vi "TestPVCam_DiskStreaming2.vi"(8 "error in":errorcluster, 10 "Exposure time [ms]":T5=20) -> (0 "error out":errorcluster)   [LabVIEW 2023, in "Photometrics Camera.lvlib"]
uses:
  Photometrics Camera.lvlib
  <userlib>/TPM LabVIEW adapter/SDK/Controls/Exposure Time.ctl
  <userlib>/TPM LabVIEW adapter/SDK/Controls/Frames To Capture.ctl
  <userlib>/TPM LabVIEW adapter/SDK/Controls/Frames Captured.ctl
  <userlib>/TPM LabVIEW adapter/SDK/Controls/Camera Description.ctl
  <userlib>/TPM LabVIEW adapter/PVCAM/PVCAM.lvclass
  <userlib>/TPM LabVIEW adapter/SDK/Controls/All Params IDs.ctl
  <userlib>/TPM LabVIEW adapter/SDK/Controls/Buffer Size.ctl
  <userlib>/TPM LabVIEW adapter/SDK/Controls/Disk Streaming Options.ctl
  <userlib>/TPM LabVIEW adapter/SDK/Controls/Disk Streaming File Name.ctl
  <userlib>/TPM LabVIEW adapter/SDK/Controls/Disk Streaming File Size.ctl
  <userlib>/TPM LabVIEW adapter/SDK/Enum params values/ENUMS/ENUM EXP RES MODES.ctl
  <userlib>/TPM LabVIEW adapter/SDK/Enum params values/RINGS/RING EXPOSURE MODES.ctl
  <userlib>/TPM LabVIEW adapter/SDK/Enum params values/ENUMS/ENUM EXPOSE OUT MODES.ctl
  <userlib>/TPM LabVIEW adapter/SDK/Controls/Acquisition Mode.ctl
  <userlib>/TPM LabVIEW adapter/Camera/Camera.lvclass
panel:
  out "Camera Description":T1
  out "Camera 0 Name":string
  out "Pixels UNS16":u16[](array[numeric])
  out "Disk Streaming Queue Count":u32
  out "Frames Captured":T2
  out "Image":T3(plugin-control)
  in  "Frames To Capture":T4=1000
  out "Disk Streaming Failed":bool
  out "Disk Streaming Dropped Frames":u64
  out "FPS":dbl
  out "Number of cameras":u32
  in  "STOP":bool
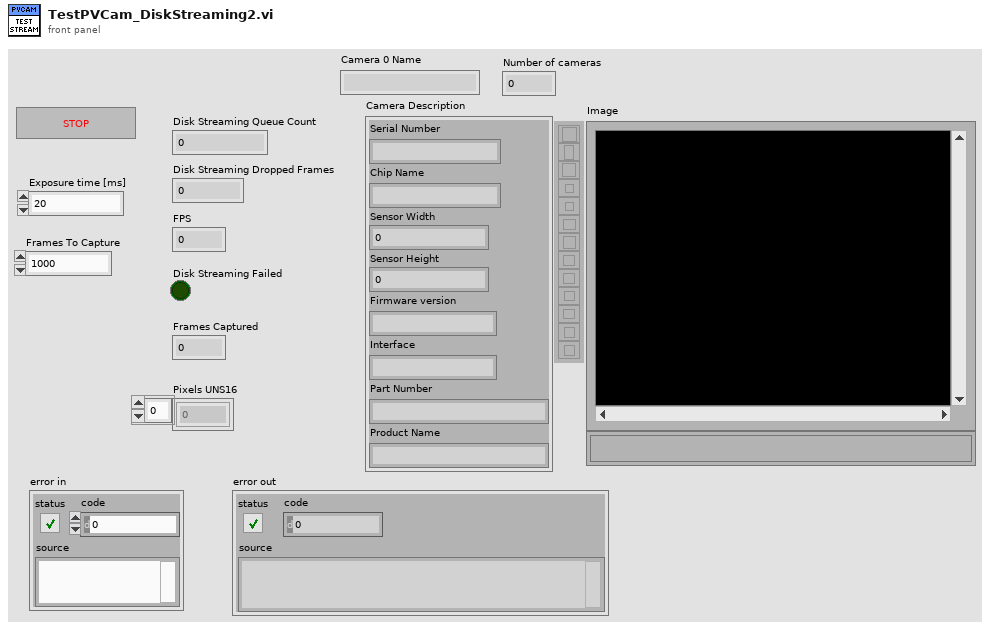
[diagram p1: front panel]
types:
  T1 = typedef "Camera Description.ctl" = cluster{"Serial Number":string, "Chip Name":string, "Sensor Width":u32, "Sensor Height":u32, "Firmware version":string, "Interface":string, "Part Number":string, "Product Name":string}
  T2 = typedef "Frames Captured.ctl" = u64
  T3 = typedef "IMAQ Image.ctl" = refnum<image>
  T4 = typedef "Frames To Capture.ctl" = u32
  T5 = typedef "Exposure Time.ctl" = u32
  T6 = typedef "ENUM EXPOSE OUT MODES.ctl" = enum32{"EXPOSE_OUT_FIRST_ROW", "EXPOSE_OUT_ALL_ROWS", "EXPOSE_OUT_ANY_ROW", "EXPOSE_OUT_ROLLING_SHUTTER", "EXPOSE_OUT_LINE_TRIGGER", "EXPOSE_OUT_GLOBAL_SHUTTER", "MAX_EXPOSE_OUT_MODE"}
  T7 = typedef "ENUM EXP RES MODES.ctl" = enum32{"EXP_RES_ONE_MILLISEC", "EXP_RES_ONE_MICROSEC", "EXP_RES_ONE_SEC"}
  T8 = typedef "Disk Streaming Options.ctl" = cluster{"Disk Streaming File Name":T9, "Path":path, "File Format":enum32{"RAW", "TIFF"}, "File Size":T10, "Big TIFF required":bool}
  T9 = typedef "Disk Streaming File Name.ctl" = string
  T10 = typedef "Disk Streaming File Size.ctl" = u64
  T11 = typedef "Buffer Size.ctl" = u32
  T12 = typedef "Acquisition Mode.ctl" = enum16{"Sequence", "Live"}
  T13 = typedef "RING EXPOSURE MODES.ctl" = u32
  T14 = typedef "All Params IDs.ctl" = i32
  T15 = typedef "Acquisition Status.ctl" = enum32{"Idle", "Starting", "Acquiring", "Stopping"}
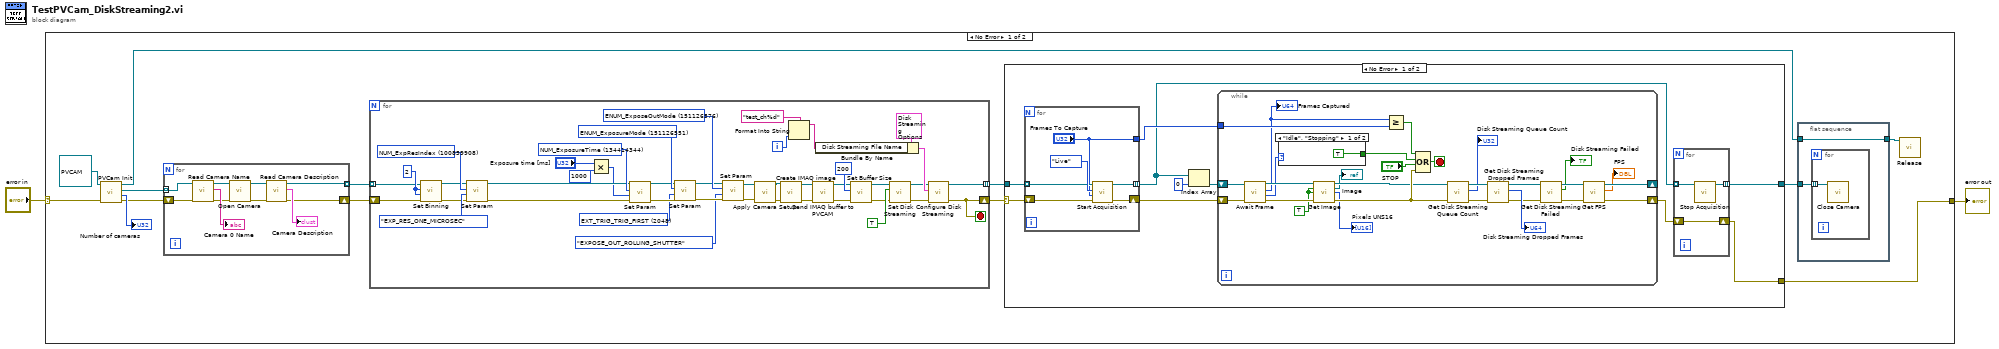
[diagram p0: block diagram]
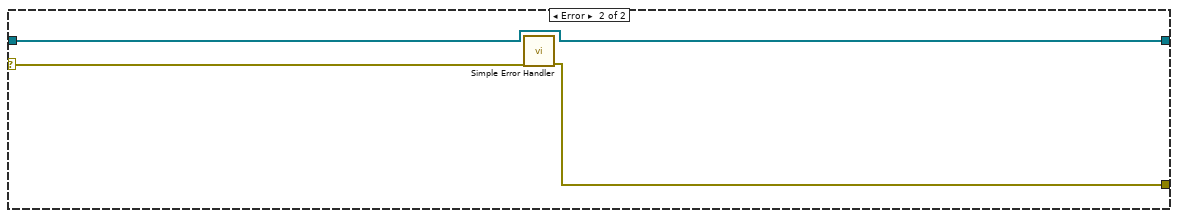
[diagram p3: hidden frame]
diagram:
  n1 = case shown="No Error" "error in" {
    selector: "error in" -> [w14 w122]
    tunnel: [w3 w122] -> w2
    frame No Error {
      n2 = call <userlib>:"PVCam Init.vi"("error in (no error)"=w14, "PVCAM In"=refnum<class "PVCAM.lvclass"> refnum ("PVCAM.lvclass")) -> ("error out"=w12:errorcluster, "Number of cameras"=→"Number of cameras":u32, "Cameras"=w8:refnum<class "Camera.lvclass">[], "PVCAM Out"=w5:refnum<class "PVCAM.lvclass">)  [unwired: 6 in]
      n3 = for {
        shift-right: [w20] -> w11
        shift-left: w12 -> [w22]
        tunnel: [w21] -> w10 mode=indexing
        tunnel: w8 -> [w19] mode=indexing
        n4 = call <userlib>:"Read Camera Name.vi"("error in (no error)"=w22, "Camera in"=w19) -> ("error out"=w26:errorcluster, "Camera Name"=→"Camera 0 Name":string, "Camera out"=w27:refnum<class "Camera.lvclass">)  [unwired: 7 in]
        n5 = call <userlib>:"Open Camera.vi"("error in (no error)"=w26, "Camera in"=w27) -> ("error out"=w25:errorcluster, "Camera out"=w24:refnum<class "Camera.lvclass">)  [unwired: 8 in]
        n6 = call-dynamic "Read Camera Description.vi"("error in (no error)"=w25, "Camera in"=w24) -> ("error out"=w20:errorcluster, "Camera Description"=→"Camera Description":T1, "Camera out"=w21:refnum<class "Camera.lvclass">)  [unwired: 7 in]
      }
      n7 = for {
        tunnel: [w59] -> w7 mode=indexing
        shift-right: [w33] -> w6
        shift-left: w11 -> [w35]
        tunnel: w10 -> [w36] mode=indexing
        i -> [w34]
        stop <- w33 stop-if-true
        w41 = T13 2048 items=["TIMED_MODE"=0, "STROBED_MODE"=1, "BULB_MODE"=2, "TRIGGER_FIRST_MODE"=3, "FLASH_MODE"=4, "VARIABLE_TIMED_MODE"=5, "INT_STROBE_MODE"=6, "MAX_EXPOSE_MODE"=7, "EXT_TRIG_INTERNAL"=1792, "EXT_TRIG_TRIG_FIRST"=2048, "EXT_TRIG_EDGE_RISING"=2304, "EXT_TRIG_LEVEL"=2560, "EXT_TRIG_SOFTWARE_FIRST"=2816, "EXT_TRIG_SOFTWARE_EDGE"=3072, "EXT_TRIG_LEVEL_OVERLAP"=3328, "EXT_TRIG_LEVEL_PULSED"=3584] ("RING Exposure Modes")
        w46 = T14 151126576 items=["BOOL_BofEofClr"=184745991, "BOOL_CentroidsEnabled"=184746154, "BOOL_CircBuffer"=184746283, "BOOL_FrameCapable"=184680957, "BOOL_GainMultEnable"=184680989, "BOOL_MetadataEnabled"=184746152, "BOOL_MetadataResetTimestamp"=184746160, "BOOL_ScanDirectionReset"=184746236, "BOOL_SmartStreamModeEnabled"=184681148, "ENUM_BinningPar"=151191718, "ENUM_BinningSer"=151191717, "ENUM_BofEofEnable"=151191557, "ENUM_CamInterfaceMode"=150994955, "ENUM_CamInterfaceType"=150994954, "ENUM_CentroidsBgCount"=151191726, "ENUM_CentroidsMode"=151191725, "ENUM_ClearMode"=151126539, "ENUM_ColorMode"=151126520, "ENUM_CoolingMode"=151126230, "ENUM_ExpRes"=151191554, "ENUM_ExposeOutMode"=151126576, "ENUM_ExposureMode"=151126551, "ENUM_FanSpeedSetpoint"=151126726, "ENUM_FrameFlip"=151126273, "ENUM_FrameRotate"=151126272, "ENUM_ImageCompression"=151126265, "ENUM_ImageFormat"=151126264, "ENUM_IoDirection"=151126545, "ENUM_IoType"=151126544, "ENUM_MppCapable"=151126240, "ENUM_PMode"=151126540, "ENUM_ReadoutPort"=151126263, "ENUM_ScanDirection"=151191803, "ENUM_ScanMode"=151191802, "ENUM_ShtrOpenMode"=151126537, "ENUM_ShtrStatus"=151126538, "ENUM_TrigTabSignal"=151191732, "NUM_ActualGain"=100794912, "NUM_AdcOffset"=16908483, "NUM_BitDepth"=16908799, "NUM_BofEofCount"=117637126, "NUM_CamFwVersion"=100794900, "NUM_CentroidsCount"=100860076, "NUM_CentroidsRadius"=100860075, "NUM_CentroidsThreshold"=117637295, "NUM_ClearCycles"=100794465, "NUM_ClearingTime"=268566708, "NUM_DdInfoLength"=16777217, "NUM_DdRetries"=100663299, "NUM_DdTimeout"=100663300, "NUM_DdVersion"=100663298, "NUM_ExpResIndex"=100859908, "NUM_ExpTime"=100859905, "NUM_ExposureTime"=134414344, "NUM_FrameBufferSize"=134414636, "NUM_FwellCapacity"=117572090, "NUM_GainIndex"=16908800, "NUM_GainMultFactor"=100794905, "NUM_IoAddr"=100794895, "NUM_IoBitDepth"=100794899, "NUM_IoState"=67240466, "NUM_LastMuxedSignal"=84082869, "NUM_ParSize"=100794425, "NUM_PciFwVersion"=100794902, "NUM_PixParDist"=100794868, "NUM_PixParSize"=100794431, "NUM_PixSerDist"=100794869, "NUM_PixSerSize"=100794430, "NUM_PixTime"=100794884, "NUM_PostTriggerDelay"=268566709, "NUM_Postmask"=100794422, "NUM_Postscan"=100794424, "NUM_PreTriggerDelay"=268566710, "NUM_PreampDelay"=100794870, "NUM_PreampOffControl"=117572091, "NUM_Premask"=100794421, "NUM_Prescan"=100794423, "NUM_ReadoutTime"=67240115, "NUM_RoiCount"=100860073, "NUM_SP_PpIndex"=16908831, "NUM_SP_PpParamIndex"=16908833, "NUM_ScanLineDelay"=100860157, "NUM_ScanLineTime"=268632318, "NUM_ScanWidth"=100860159, "NUM_SerSize"=100794426, "NUM_ShtrCloseDelay"=100794887, "NUM_ShtrOpenDelay"=100794888, "NUM_SmartStreamMode"=100795069, "NUM_SpdtabIndex"=16908801, "NUM_SummingWell"=184680953, "NUM_Temp"=16908813, "NUM_TempSetpoint"=16908814, "PP_PpFeatId"=100794917, "PP_PpParam"=117572131, "PP_PpParamId"=100794918, "PP_ReadNoise"=100794916, "SS_SmartStreamDlyParams"=235012799, "SS_SmartStreamModeExpParams"=235012798, "STR_CamSystemsInfo"=218235416, "STR_CameraPartNumber"=218235013, "STR_ChipName"=218235009, "STR_DdInfo"=218103813, "STR_GainName"=218235394, "STR_HeadSerNumAlpha"=218235413, "STR_PpFeatName"=218235422, "STR_PpParamName"=218235426, "STR_ProductName"=218235012, "STR_SystemName"=218235010, "STR_VendorName"=218235011] ("PVCAM Param IDs")
        w47 = T14 151126551 items=["BOOL_BofEofClr"=184745991, "BOOL_CentroidsEnabled"=184746154, "BOOL_CircBuffer"=184746283, "BOOL_FrameCapable"=184680957, "BOOL_GainMultEnable"=184680989, "BOOL_MetadataEnabled"=184746152, "BOOL_MetadataResetTimestamp"=184746160, "BOOL_ScanDirectionReset"=184746236, "BOOL_SmartStreamModeEnabled"=184681148, "ENUM_BinningPar"=151191718, "ENUM_BinningSer"=151191717, "ENUM_BofEofEnable"=151191557, "ENUM_CamInterfaceMode"=150994955, "ENUM_CamInterfaceType"=150994954, "ENUM_CentroidsBgCount"=151191726, "ENUM_CentroidsMode"=151191725, "ENUM_ClearMode"=151126539, "ENUM_ColorMode"=151126520, "ENUM_CoolingMode"=151126230, "ENUM_ExpRes"=151191554, "ENUM_ExposeOutMode"=151126576, "ENUM_ExposureMode"=151126551, "ENUM_FanSpeedSetpoint"=151126726, "ENUM_FrameFlip"=151126273, "ENUM_FrameRotate"=151126272, "ENUM_ImageCompression"=151126265, "ENUM_ImageFormat"=151126264, "ENUM_IoDirection"=151126545, "ENUM_IoType"=151126544, "ENUM_MppCapable"=151126240, "ENUM_PMode"=151126540, "ENUM_ReadoutPort"=151126263, "ENUM_ScanDirection"=151191803, "ENUM_ScanMode"=151191802, "ENUM_ShtrOpenMode"=151126537, "ENUM_ShtrStatus"=151126538, "ENUM_TrigTabSignal"=151191732, "NUM_ActualGain"=100794912, "NUM_AdcOffset"=16908483, "NUM_BitDepth"=16908799, "NUM_BofEofCount"=117637126, "NUM_CamFwVersion"=100794900, "NUM_CentroidsCount"=100860076, "NUM_CentroidsRadius"=100860075, "NUM_CentroidsThreshold"=117637295, "NUM_ClearCycles"=100794465, "NUM_ClearingTime"=268566708, "NUM_DdInfoLength"=16777217, "NUM_DdRetries"=100663299, "NUM_DdTimeout"=100663300, "NUM_DdVersion"=100663298, "NUM_ExpResIndex"=100859908, "NUM_ExpTime"=100859905, "NUM_ExposureTime"=134414344, "NUM_FrameBufferSize"=134414636, "NUM_FwellCapacity"=117572090, "NUM_GainIndex"=16908800, "NUM_GainMultFactor"=100794905, "NUM_IoAddr"=100794895, "NUM_IoBitDepth"=100794899, "NUM_IoState"=67240466, "NUM_LastMuxedSignal"=84082869, "NUM_ParSize"=100794425, "NUM_PciFwVersion"=100794902, "NUM_PixParDist"=100794868, "NUM_PixParSize"=100794431, "NUM_PixSerDist"=100794869, "NUM_PixSerSize"=100794430, "NUM_PixTime"=100794884, "NUM_PostTriggerDelay"=268566709, "NUM_Postmask"=100794422, "NUM_Postscan"=100794424, "NUM_PreTriggerDelay"=268566710, "NUM_PreampDelay"=100794870, "NUM_PreampOffControl"=117572091, "NUM_Premask"=100794421, "NUM_Prescan"=100794423, "NUM_ReadoutTime"=67240115, "NUM_RoiCount"=100860073, "NUM_SP_PpIndex"=16908831, "NUM_SP_PpParamIndex"=16908833, "NUM_ScanLineDelay"=100860157, "NUM_ScanLineTime"=268632318, "NUM_ScanWidth"=100860159, "NUM_SerSize"=100794426, "NUM_ShtrCloseDelay"=100794887, "NUM_ShtrOpenDelay"=100794888, "NUM_SmartStreamMode"=100795069, "NUM_SpdtabIndex"=16908801, "NUM_SummingWell"=184680953, "NUM_Temp"=16908813, "NUM_TempSetpoint"=16908814, "PP_PpFeatId"=100794917, "PP_PpParam"=117572131, "PP_PpParamId"=100794918, "PP_ReadNoise"=100794916, "SS_SmartStreamDlyParams"=235012799, "SS_SmartStreamModeExpParams"=235012798, "STR_CamSystemsInfo"=218235416, "STR_CameraPartNumber"=218235013, "STR_ChipName"=218235009, "STR_DdInfo"=218103813, "STR_GainName"=218235394, "STR_HeadSerNumAlpha"=218235413, "STR_PpFeatName"=218235422, "STR_PpParamName"=218235426, "STR_ProductName"=218235012, "STR_SystemName"=218235010, "STR_VendorName"=218235011] ("PVCAM Param IDs")
        w52 = T14 100859908 items=["BOOL_BofEofClr"=184745991, "BOOL_CentroidsEnabled"=184746154, "BOOL_CircBuffer"=184746283, "BOOL_FrameCapable"=184680957, "BOOL_GainMultEnable"=184680989, "BOOL_MetadataEnabled"=184746152, "BOOL_MetadataResetTimestamp"=184746160, "BOOL_ScanDirectionReset"=184746236, "BOOL_SmartStreamModeEnabled"=184681148, "ENUM_BinningPar"=151191718, "ENUM_BinningSer"=151191717, "ENUM_BofEofEnable"=151191557, "ENUM_CamInterfaceMode"=150994955, "ENUM_CamInterfaceType"=150994954, "ENUM_CentroidsBgCount"=151191726, "ENUM_CentroidsMode"=151191725, "ENUM_ClearMode"=151126539, "ENUM_ColorMode"=151126520, "ENUM_CoolingMode"=151126230, "ENUM_ExpRes"=151191554, "ENUM_ExposeOutMode"=151126576, "ENUM_ExposureMode"=151126551, "ENUM_FanSpeedSetpoint"=151126726, "ENUM_FrameFlip"=151126273, "ENUM_FrameRotate"=151126272, "ENUM_ImageCompression"=151126265, "ENUM_ImageFormat"=151126264, "ENUM_IoDirection"=151126545, "ENUM_IoType"=151126544, "ENUM_MppCapable"=151126240, "ENUM_PMode"=151126540, "ENUM_ReadoutPort"=151126263, "ENUM_ScanDirection"=151191803, "ENUM_ScanMode"=151191802, "ENUM_ShtrOpenMode"=151126537, "ENUM_ShtrStatus"=151126538, "ENUM_TrigTabSignal"=151191732, "NUM_ActualGain"=100794912, "NUM_AdcOffset"=16908483, "NUM_BitDepth"=16908799, "NUM_BofEofCount"=117637126, "NUM_CamFwVersion"=100794900, "NUM_CentroidsCount"=100860076, "NUM_CentroidsRadius"=100860075, "NUM_CentroidsThreshold"=117637295, "NUM_ClearCycles"=100794465, "NUM_ClearingTime"=268566708, "NUM_DdInfoLength"=16777217, "NUM_DdRetries"=100663299, "NUM_DdTimeout"=100663300, "NUM_DdVersion"=100663298, "NUM_ExpResIndex"=100859908, "NUM_ExpTime"=100859905, "NUM_ExposureTime"=134414344, "NUM_FrameBufferSize"=134414636, "NUM_FwellCapacity"=117572090, "NUM_GainIndex"=16908800, "NUM_GainMultFactor"=100794905, "NUM_IoAddr"=100794895, "NUM_IoBitDepth"=100794899, "NUM_IoState"=67240466, "NUM_LastMuxedSignal"=84082869, "NUM_ParSize"=100794425, "NUM_PciFwVersion"=100794902, "NUM_PixParDist"=100794868, "NUM_PixParSize"=100794431, "NUM_PixSerDist"=100794869, "NUM_PixSerSize"=100794430, "NUM_PixTime"=100794884, "NUM_PostTriggerDelay"=268566709, "NUM_Postmask"=100794422, "NUM_Postscan"=100794424, "NUM_PreTriggerDelay"=268566710, "NUM_PreampDelay"=100794870, "NUM_PreampOffControl"=117572091, "NUM_Premask"=100794421, "NUM_Prescan"=100794423, "NUM_ReadoutTime"=67240115, "NUM_RoiCount"=100860073, "NUM_SP_PpIndex"=16908831, "NUM_SP_PpParamIndex"=16908833, "NUM_ScanLineDelay"=100860157, "NUM_ScanLineTime"=268632318, "NUM_ScanWidth"=100860159, "NUM_SerSize"=100794426, "NUM_ShtrCloseDelay"=100794887, "NUM_ShtrOpenDelay"=100794888, "NUM_SmartStreamMode"=100795069, "NUM_SpdtabIndex"=16908801, "NUM_SummingWell"=184680953, "NUM_Temp"=16908813, "NUM_TempSetpoint"=16908814, "PP_PpFeatId"=100794917, "PP_PpParam"=117572131, "PP_PpParamId"=100794918, "PP_ReadNoise"=100794916, "SS_SmartStreamDlyParams"=235012799, "SS_SmartStreamModeExpParams"=235012798, "STR_CamSystemsInfo"=218235416, "STR_CameraPartNumber"=218235013, "STR_ChipName"=218235009, "STR_DdInfo"=218103813, "STR_GainName"=218235394, "STR_HeadSerNumAlpha"=218235413, "STR_PpFeatName"=218235422, "STR_PpParamName"=218235426, "STR_ProductName"=218235012, "STR_SystemName"=218235010, "STR_VendorName"=218235011] ("PVCAM Param IDs")
        w54 = u16 2 ("Binning X")
        w70 = T14 134414344 items=["BOOL_BofEofClr"=184745991, "BOOL_CentroidsEnabled"=184746154, "BOOL_CircBuffer"=184746283, "BOOL_FrameCapable"=184680957, "BOOL_GainMultEnable"=184680989, "BOOL_MetadataEnabled"=184746152, "BOOL_MetadataResetTimestamp"=184746160, "BOOL_ScanDirectionReset"=184746236, "BOOL_SmartStreamModeEnabled"=184681148, "ENUM_BinningPar"=151191718, "ENUM_BinningSer"=151191717, "ENUM_BofEofEnable"=151191557, "ENUM_CamInterfaceMode"=150994955, "ENUM_CamInterfaceType"=150994954, "ENUM_CentroidsBgCount"=151191726, "ENUM_CentroidsMode"=151191725, "ENUM_ClearMode"=151126539, "ENUM_ColorMode"=151126520, "ENUM_CoolingMode"=151126230, "ENUM_ExpRes"=151191554, "ENUM_ExposeOutMode"=151126576, "ENUM_ExposureMode"=151126551, "ENUM_FanSpeedSetpoint"=151126726, "ENUM_FrameFlip"=151126273, "ENUM_FrameRotate"=151126272, "ENUM_ImageCompression"=151126265, "ENUM_ImageFormat"=151126264, "ENUM_IoDirection"=151126545, "ENUM_IoType"=151126544, "ENUM_MppCapable"=151126240, "ENUM_PMode"=151126540, "ENUM_ReadoutPort"=151126263, "ENUM_ScanDirection"=151191803, "ENUM_ScanMode"=151191802, "ENUM_ShtrOpenMode"=151126537, "ENUM_ShtrStatus"=151126538, "ENUM_TrigTabSignal"=151191732, "NUM_ActualGain"=100794912, "NUM_AdcOffset"=16908483, "NUM_BitDepth"=16908799, "NUM_BofEofCount"=117637126, "NUM_CamFwVersion"=100794900, "NUM_CentroidsCount"=100860076, "NUM_CentroidsRadius"=100860075, "NUM_CentroidsThreshold"=117637295, "NUM_ClearCycles"=100794465, "NUM_ClearingTime"=268566708, "NUM_DdInfoLength"=16777217, "NUM_DdRetries"=100663299, "NUM_DdTimeout"=100663300, "NUM_DdVersion"=100663298, "NUM_ExpResIndex"=100859908, "NUM_ExpTime"=100859905, "NUM_ExposureTime"=134414344, "NUM_FrameBufferSize"=134414636, "NUM_FwellCapacity"=117572090, "NUM_GainIndex"=16908800, "NUM_GainMultFactor"=100794905, "NUM_IoAddr"=100794895, "NUM_IoBitDepth"=100794899, "NUM_IoState"=67240466, "NUM_LastMuxedSignal"=84082869, "NUM_ParSize"=100794425, "NUM_PciFwVersion"=100794902, "NUM_PixParDist"=100794868, "NUM_PixParSize"=100794431, "NUM_PixSerDist"=100794869, "NUM_PixSerSize"=100794430, "NUM_PixTime"=100794884, "NUM_PostTriggerDelay"=268566709, "NUM_Postmask"=100794422, "NUM_Postscan"=100794424, "NUM_PreTriggerDelay"=268566710, "NUM_PreampDelay"=100794870, "NUM_PreampOffControl"=117572091, "NUM_Premask"=100794421, "NUM_Prescan"=100794423, "NUM_ReadoutTime"=67240115, "NUM_RoiCount"=100860073, "NUM_SP_PpIndex"=16908831, "NUM_SP_PpParamIndex"=16908833, "NUM_ScanLineDelay"=100860157, "NUM_ScanLineTime"=268632318, "NUM_ScanWidth"=100860159, "NUM_SerSize"=100794426, "NUM_ShtrCloseDelay"=100794887, "NUM_ShtrOpenDelay"=100794888, "NUM_SmartStreamMode"=100795069, "NUM_SpdtabIndex"=16908801, "NUM_SummingWell"=184680953, "NUM_Temp"=16908813, "NUM_TempSetpoint"=16908814, "PP_PpFeatId"=100794917, "PP_PpParam"=117572131, "PP_PpParamId"=100794918, "PP_ReadNoise"=100794916, "SS_SmartStreamDlyParams"=235012799, "SS_SmartStreamModeExpParams"=235012798, "STR_CamSystemsInfo"=218235416, "STR_CameraPartNumber"=218235013, "STR_ChipName"=218235009, "STR_DdInfo"=218103813, "STR_GainName"=218235394, "STR_HeadSerNumAlpha"=218235413, "STR_PpFeatName"=218235422, "STR_PpParamName"=218235426, "STR_ProductName"=218235012, "STR_SystemName"=218235010, "STR_VendorName"=218235011] ("PVCAM Param IDs")
        n8 = call <userlib>:"Set Binning.vi"("error in (no error)"=w35, "Binning Y"=w54, "Binning X"=w54, "Camera in"=w36) -> ("error out"=w50:errorcluster, "Camera out"=w51:refnum<class "Camera.lvclass">)  [unwired: 6 in]
        n9 = call <userlib>:"Set Param.vi"("error in (no error)"=w50, "Parameter value"=ENUM_EXP_RES_MODES."EXP_RES_ONE_MICROSEC" ("ENUM Exp Res Modes"), "PVCAM Param IDs"=w52, "Camera In"=w51) -> ("error out"=w48:errorcluster, "Camera Out"=w49:refnum<class "Camera.lvclass">)  [unwired: 6 in]
        n10 = Multiply(x="Exposure time [ms]", y=T5 1000) -> (x*y=w37:T5)
        n11 = call <userlib>:"Set Param.vi"("error in (no error)"=w48, "Parameter value"=w37, "PVCAM Param IDs"=w70, "Camera In"=w49) -> ("error out"=w42:errorcluster, "Camera Out"=w43:refnum<class "Camera.lvclass">)  [unwired: 6 in]
        n12 = call <userlib>:"Set Param.vi"("error in (no error)"=w42, "Parameter value"=w41, "PVCAM Param IDs"=w47, "Camera In"=w43) -> ("error out"=w45:errorcluster, "Camera Out"=w44:refnum<class "Camera.lvclass">)  [unwired: 6 in]
        n13 = call <userlib>:"Set Param.vi"("error in (no error)"=w45, "Parameter value"=ENUM_EXPOSE_OUT_MODES."EXPOSE_OUT_ROLLING_SHUTTER" ("ENUM Expose Out Modes"), "PVCAM Param IDs"=w46, "Camera In"=w44) -> ("error out"=w31:errorcluster, "Camera Out"=w32:refnum<class "Camera.lvclass">)  [unwired: 6 in]
        n14 = call <userlib>:"Apply Camera Setup.vi"("error in (no error)"=w31, "Camera in"=w32) -> ("error out"=w29:errorcluster, "Camera out"=w30:refnum<class "Camera.lvclass">)  [unwired: 8 in]
        n15 = call <userlib>:"Create IMAQ image.vi"("error in (no error)"=w29, "Camera in"=w30) -> ("error out"=w58:errorcluster, "Camera out"=w57:refnum<class "Camera.lvclass">)  [unwired: 8 in]
        n16 = Format Into String(format string="test_ch%d", w34) -> (resulting string=w67:string)  [unwired: 2 in, 1 out]
        n17 = call <userlib>:"Send IMAQ buffer to PVCAM.vi"("error in (no error)"=w58, "Camera in"=w57) -> ("error out"=w55:errorcluster, "Camera out"=w56:refnum<class "Camera.lvclass">)  [unwired: 8 in]
        n18 = Bundle By Name(cluster=T8 {"Disk Streaming File Name"="test", "Path"=path "E:/", "File Format"=enum."RAW", "File Size"=1000000000000, "Big TIFF required"=FALSE} ("Disk Streaming Options"), "Disk Streaming File Name"=w67) -> (w66:T8)
        n19 = call <userlib>:"Set Buffer Size.vi"("error in (no error)"=w55, "Buffer Size Frames"=T11 200, "Camera in"=w56) -> ("error out"=w61:errorcluster, "Camera out"=w63:refnum<class "Camera.lvclass">)  [unwired: 7 in]
        n20 = call <userlib>:"Set Disk Streaming.vi"("error in (no error)"=w61, "Enable/Disable streaming"=TRUE, "Camera in"=w63) -> ("error out"=w62:errorcluster, "Camera out"=w60:refnum<class "Camera.lvclass">)  [unwired: 7 in]
        n21 = call <userlib>:"Configure Disk Streaming.vi"("error in (no error)"=w62, "Disk Streaming Options"=w66, "Camera in"=w60) -> ("error out"=w33:errorcluster, "Camera out"=w59:refnum<class "Camera.lvclass">)  [unwired: 7 in]
      }
      n22 = case shown="No Error" w6 {
        selector: w6 -> [w73 w121]
        tunnel: [w80 w120] -> w9
        tunnel: w7 -> [w79 w120]
        tunnel: [w71 w119] -> w3
        frame No Error {
          n23 = for {
            tunnel: w79 -> [w87] mode=indexing
            shift-right: [w86] -> w77
            shift-left: w73 -> [w88]
            tunnel: ["Frames To Capture"] -> w78
            tunnel: [w84] -> w75 mode=indexing
            n24 = call <userlib>:"Start Acquisition.vi"("error in (no error)"=w88, "Frames To Capture"="Frames To Capture", "Acquisition Mode"=Acquisition_Mode."Live", "Camera in"=w87) -> ("error out"=w86:errorcluster, "Camera out"=w84:refnum<class "Camera.lvclass">)  [unwired: 6 in]
          }
          n25 = Index Array(array=w75, index=0) -> (element=w76:refnum<class "Camera.lvclass">)
          n26 = while {
            shift-right: [w108] -> _
            shift-left: w76 -> [w116]
            shift-right: [w109] -> w72
            shift-left: w77 -> [w117]
            tunnel: w78 -> [w95]
            stop <- w112 stop-if-true
            w91 = TRUE ("Get Image (T)")
            n27 = call <userlib>:"Await Frame.vi"("error in (no error)"=w117, "Camera in"=w116) -> ("error out"=w115:errorcluster, "Acquisition Status"=w113:T15, "Frames Captured"=w94:T2, "Camera out"=w114:refnum<class "Camera.lvclass">)  [unwired: 6 in]
            "Frames Captured" <- w94
            n28 = case shown="\"Idle\", \"Stopping\"" w113 {
              tunnel: [TRUE ("value") _] -> w111
              frame "Idle", "Stopping" {
              }
              frame Default {
              }
            }
            n29 = call <userlib>:"Get Image.vi"("Camera in"=w114, "Get Image (T)"=w91, "Get Pixel Array (F)"=w91, "error in (no error)"=w115) -> ("Camera out"=w103:refnum<class "Camera.lvclass">, "IMAQ image"=→"Image":T3, "Pixels UNS16"=→"Pixels UNS16":u16[], "error out"=w106:errorcluster)  [unwired: 6 in, 2 out]
            n30 = Greater Or Equal?(x=w94, y=w95) -> (x >= y?=w93:bool)
            n31 = Compound Arithmetic op=OR(w93, w111, "STOP", w106) -> (w112:bool)
            n32 = call <userlib>:"Get Disk Streaming Queue Count.vi"("error in (no error)"=w106, "Camera in"=w103) -> ("error out"=w105:errorcluster, "Disk Streaming Queue Count"=→"Disk Streaming Queue Count":u32, "Camera out"=w104:refnum<class "Camera.lvclass">)  [unwired: 7 in]
            n33 = call <userlib>:"Get Disk Streaming Dropped Frames.vi"("error in (no error)"=w105, "Camera in"=w104) -> ("error out"=w101:errorcluster, "Disk Streaming Dropped Frames"=→"Disk Streaming Dropped Frames":u64, "Camera out"=w99:refnum<class "Camera.lvclass">)  [unwired: 7 in]
            n34 = call <userlib>:"Get Disk Streaming Failed.vi"("error in (no error)"=w101, "Camera in"=w99) -> ("error out"=w100:errorcluster, "Disk Streaming Failed"=→"Disk Streaming Failed":bool, "Camera out"=w98:refnum<class "Camera.lvclass">)  [unwired: 7 in]
            n35 = call <userlib>:"Get FPS.vi"("error in (no error)"=w100, "Camera in"=w98) -> ("error out"=w109:errorcluster, "FPS"=→"FPS":dbl, "Camera out"=w108:refnum<class "Camera.lvclass">)  [unwired: 7 in]
          }
          n36 = for {
            tunnel: w75 -> [w83] mode=indexing
            tunnel: [w82] -> w80 mode=indexing
            shift-right: [w81] -> w71
            shift-left: w72 -> [w81]
            n37 = call <userlib>:"Stop Acquisition.vi"("Camera in"=w83) -> ("Camera out"=w82:refnum<class "Camera.lvclass">)  [unwired: 9 in, 1 out]
          }
        }
        frame Error {
          n38 = call <vilib>:"Simple Error Handler.vi"("error in (no error)"=w121) -> ("error out"=w119:errorcluster)  [unwired: 4 in, 4 out]
        }
      }
      n39 = flat-sequence {
        tunnel: w9 -> [w17]
        tunnel: w5 -> [w16]
        tunnel: [w16] -> w4
        frame #0 {
          n40 = for {
            tunnel: w17 -> [w18] mode=indexing
            n41 = call <userlib>:"Close Camera.vi"("Camera in"=w18) -> ()  [unwired: 9 in, 2 out]
          }
        }
      }
      n42 = call <userlib>:"Release.vi"("PVCAM in"=w4) -> ()  [unwired: 9 in, 2 out]
    }
    frame Error {
    }
  }
  "error out" <- w2
